vi "Send Created.vi"(8 "Alias":string, 9 "Is Priority":bool, 10 "Msg":refnum<class "Msg.lvclass">, 11 "Base Actor in":refnum<class "Base Actor.lvclass">) -> (3 "Base Actor out":refnum<class "Base Actor.lvclass">)   [LabVIEW 2020, in "jettl.lvlib" / "Actor.lvlib" / "Base Actor.lvclass"]
uses:
  Base Actor.lvclass
  Msg/Msg.lvclass
  Relation.ctl
  Attributes/Attributes/Attributes.lvclass
  Actor.lvlib
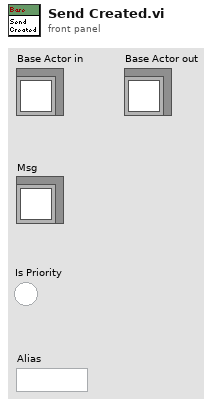
[diagram p1: front panel]
types:
  T1 = typedef "jettl.lvlib/Actor.lvlib/Map of Created Attributes.ctl" = map{string, refnum<class "Attributes.lvclass">}
  T2 = typedef "jettl.lvlib/Actor.lvlib/Relation.ctl" = enum16{"Self", "Creator", "Created"}
  T3 = typedef "jettl.lvlib/Actor.lvlib/Msgs.ctl" = set{refnum<class "Msg.lvclass">}
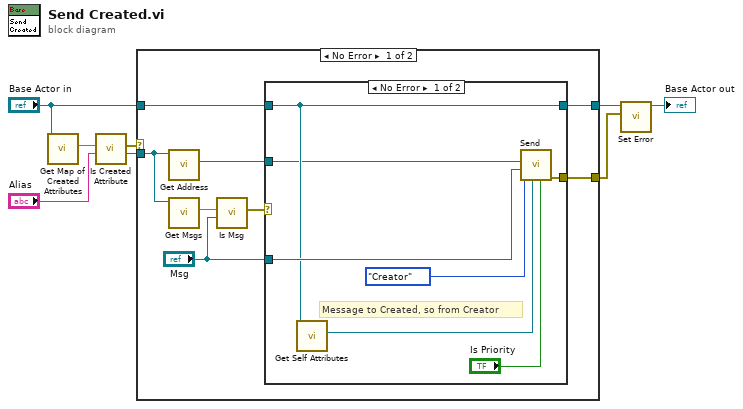
[diagram p0: block diagram]
diagram:
  n1 = call-dynamic "Get Map of Created Attributes.vi"("Base Actor in"="Base Actor in") -> ("Map of Created Attributes"=w4:T1)  [unwired: 10 in]
  n2 = call "Is Created Attribute.vi"("Alias"="Alias", "Map of Created Attributes"=w4) -> ("Created Attributes"=w1:refnum<class "Attributes.lvclass">, "Error"=w2:errorcluster)  [unwired: 8 in]
  n3 = case shown="No Error" w2 {
    selector: w2 -> [_ w26]
    tunnel: [w16 w27] -> w7
    tunnel: "Base Actor in" -> [w15 w27]
    tunnel: [w14 w26] -> w5
    tunnel: w1 -> [w10 _]
    frame No Error {
      n4 = call-dynamic "Get Address.vi"("Attributes in"=w10) -> ("Address"=w11:refnum<user-event>)  [unwired: 10 in]
      n5 = call-dynamic "Get Msgs.vi"("Attributes in"=w10) -> ("Msgs"=w13:T3)  [unwired: 10 in]
      n6 = call "Is Msg.vi"("Msg"="Msg", "Msgs"=w13) -> ("Error"=w12:errorcluster)  [unwired: 9 in]
      n7 = case shown="No Error" w12 {
        selector: w12 -> [_ w24]
        tunnel: w15 -> [w19 w25]
        tunnel: [w19 w25] -> w16
        tunnel: "Msg" -> [w23 _]
        tunnel: [w18 w24] -> w14
        tunnel: w11 -> [w17 _]
        frame No Error {
          # "Message to Created, so from Creator"
          n8 = call-dynamic "Get Self Attributes.vi"("Base Actor in"=w19) -> ("Self Attributes"=w21:refnum<class "Attributes.lvclass">)  [unwired: 10 in]
          n9 = call "Send.vi"("Is Priority"="Is Priority", "Self Attributes"=w21, "Relation"=Relation."Creator", "Msg"=w23, "Address"=w17) -> ("Error"=w18:errorcluster)  [unwired: 6 in]
        }
        frame Error {
        }
      }
    }
    frame Error {
    }
  }
  n10 = call-dynamic "Set Error.vi"("Error"=w5, "Base Actor in"=w7) -> ("Base Actor out"=→"Base Actor out":refnum<class "Base Actor.lvclass">)  [unwired: 9 in]
